vi "KeyBoardSimulation.vi"() -> ()   [LabVIEW 2016, in "DronaTest.lvlib" / "test_ValueSignal.lvlib"]
uses:
  test_ValueSignal.lvlib
  Helper/HelperVI-keyboardsimulation.vi
  main/apis/Setup/GetVI/GetVIByPath.vi
  main/apis/Assert/AssertControlValue/Equal.vi
  main/apis/Assert/AssertControlValue/True.vi
  main/apis/Stimulus/ValueSignal/ValueSignalByPathString.vi
  main/Drona.lvlib
  main/apis/Setup/GetVI/GetVI.lvlib
  main/apis/Assert/AssertControlValue/AssertControlValue.lvlib
  <vilib>/addons/_JKI Toolkits/Caraya/classes/Test/Test.lvclass
  main/apis/Stimulus/ValueSignal/ValueSignal.lvlib
panel:
  out "error out":errorcluster
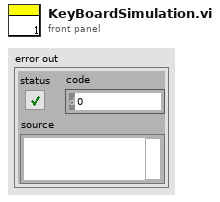
[diagram p1: front panel]
types:
  T1 = cluster{" Key":u8, "Action":enum16{"Press", "Up", "Down"}, "Delay (ms)":u32}[]
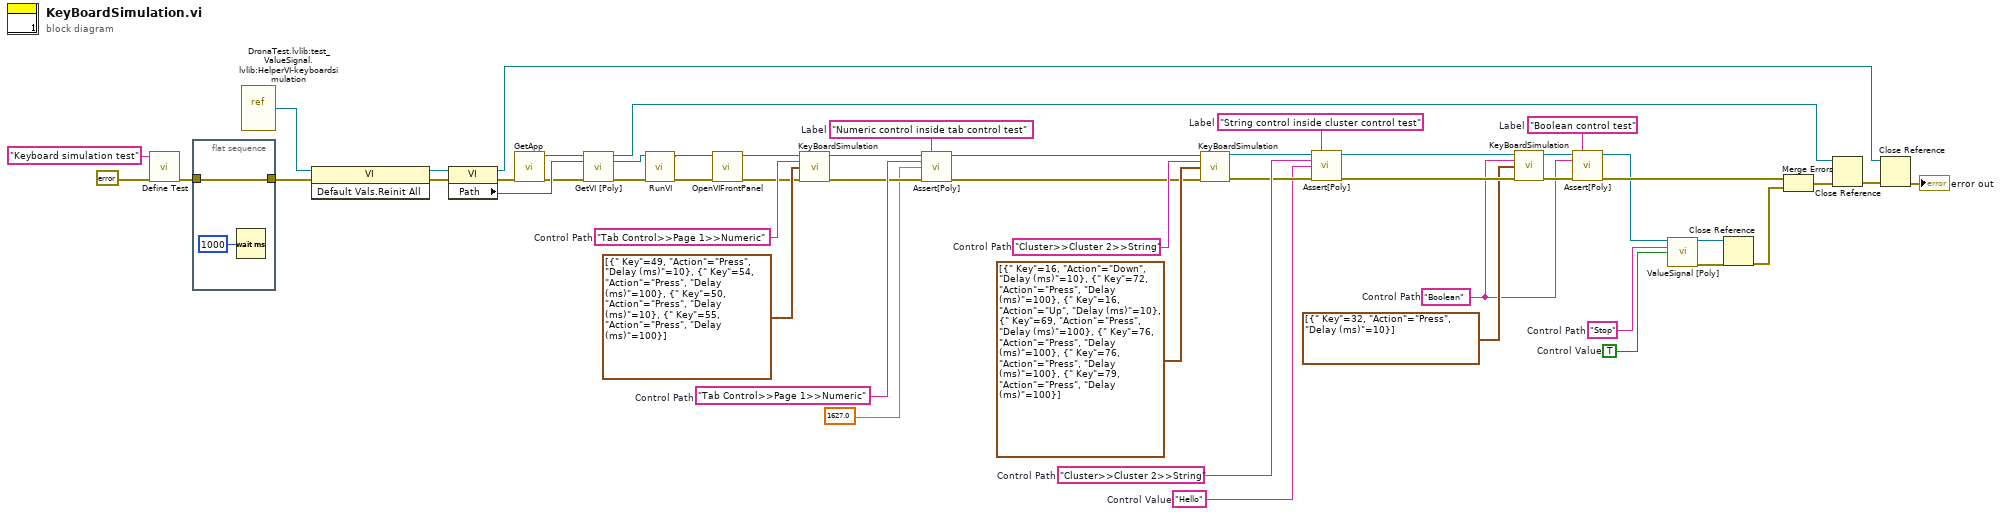
[diagram p0: block diagram]
diagram:
  w1 = "Boolean control test"  # Label
  w2 = "Boolean"  # Control Path
  w27 = TRUE  # Control Value
  w28 = "Stop"  # Control Path
  w30 = "Hello"  # Control Value
  w35 = "String control inside cluster control test"  # Label
  w36 = "Cluster>>Cluster 2>>String"  # Control Path
  w38 = "Tab Control>>Page 1>>Numeric"  # Control Path
  w43 = "Numeric control inside tab control test"  # Label
  w44 = "Tab Control>>Page 1>>Numeric"  # Control Path
  w32 = "Cluster>>Cluster 2>>String"  # Control Path
  n1 = call <vilib>:"Define Test.vi"("error in (no error)"=errorcluster {"status"=FALSE, "code"=0, "source"=""}, "Label (VI Title)"="Keyboard simulation test") -> ("error out"=w15:errorcluster)  [unwired: 9 in]
  n2 = flat-sequence {
    tunnel: w15 -> [w54]
    tunnel: [w54] -> w14
    frame #0 {
      n3 = Wait (ms)(milliseconds to wait=u32 1000) -> ()  [unwired: 1 out]
    }
  }
  n4 = vi-ref "DronaTest.lvlib:test_ValueSignal.lvlib:HelperVI-keyboardsimulation.vi"() -> (w18:refnum<vi>)
  n5 = invoke class="VI" method="Default Vals.Reinit All"(reference=w18, error in=w14) -> (reference out=w19:refnum<vi>, error out=w20:errorcluster)  [unwired: 1 in, 1 out]
  n6 = property on="Property Node" class="VI"(reference=w19, error in=w20) -> (reference out=w45:refnum<vi>, error out=w49:errorcluster, "Path"=w48:path)
  n7 = call "GetApp.vi"("error in (no error)"=w49) -> ("Application Ref"=w50:refnum<vi>, "error out"=w47:errorcluster)  [unwired: 13 in]
  n8 = call-poly "GetVI [Poly].vi"("Application Ref in"=w50, "VI Path"=w48, "error in (no error)"=w47) -> ("Application Ref out"=w46:refnum<vi>, "VI Reference"=w41:refnum<vi>, "error out"=w42:errorcluster)  [unwired: 10 in]
  n9 = call "RunVI.vi"("VI Reference In"=w41, "error in"=w42) -> ("VI Reference Out"=w12:refnum<vi>, "error out"=w13:errorcluster)  [unwired: 12 in]
  n10 = call "OpenVIFrontPanel.vi"("VI Reference In"=w12, "error in"=w13) -> ("VI Reference Out"=w11:refnum<vi>, "error out"=w10:errorcluster)  [unwired: 12 in]
  n11 = call "KeyBoardSimulation.vi"("VI Reference In"=w11, "Control Path"=w38, "Key Array"=T1 [{" Key"=49, "Action"=enum."Press", "Delay (ms)"=10}, {" Key"=54, "Action"=enum."Press", "Delay (ms)"=100}, {" Key"=50, "Action"=enum."Press", "Delay (ms)"=10}, {" Key"=55, "Action"=enum."Press", "Delay (ms)"=100}], "error In"=w10) -> ("VI Reference Out"=w39:refnum<vi>, "error IO"=w40:errorcluster)  [unwired: 10 in]
  n12 = call-poly "Assert[Poly].vi"("VI Reference In"=w39, "Label"=w43, "Control Path"=w44, "Control Value"=1627.0, "Error In"=w40) -> ("VI Reference Out"=w24:refnum<vi>, "Error Out"=w25:errorcluster)  [unwired: 9 in]
  n13 = call "KeyBoardSimulation.vi"("VI Reference In"=w24, "Control Path"=w32, "Key Array"=T1 [{" Key"=16, "Action"=enum."Down", "Delay (ms)"=10}, {" Key"=72, "Action"=enum."Press", "Delay (ms)"=100}, {" Key"=16, "Action"=enum."Up", "Delay (ms)"=10}, {" Key"=69, "Action"=enum."Press", "Delay (ms)"=100}, {" Key"=76, "Action"=enum."Press", "Delay (ms)"=100}, {" Key"=76, "Action"=enum."Press", "Delay (ms)"=100}, {" Key"=79, "Action"=enum."Press", "Delay (ms)"=100}], "error In"=w25) -> ("VI Reference Out"=w33:refnum<vi>, "error IO"=w34:errorcluster)  [unwired: 10 in]
  n14 = call-poly "Assert[Poly].vi"("VI Reference In"=w33, "Label"=w35, "Control Path"=w36, "Control Value"=w30, "Error In"=w34) -> ("VI Reference Out"=w8:refnum<vi>, "Error Out"=w9:errorcluster)  [unwired: 9 in]
  n15 = call "KeyBoardSimulation.vi"("VI Reference In"=w8, "Control Path"=w2, "Key Array"=T1 [{" Key"=32, "Action"=enum."Press", "Delay (ms)"=10}], "error In"=w9) -> ("VI Reference Out"=w4:refnum<vi>, "error IO"=w6:errorcluster)  [unwired: 10 in]
  n16 = call-poly "Assert[Poly].vi"("VI Reference In"=w4, "Label"=w1, "Control Path"=w2, "Error In"=w6) -> ("VI Reference Out"=w3:refnum<vi>, "Error Out"=w5:errorcluster)  [unwired: 10 in]
  n17 = call-poly "ValueSignal [Poly].vi"("VI Reference In"=w3, "Control Path"=w28, "Value (Signaling)"=w27) -> ("VI Reference Out"=w26:refnum<vi>, "error out"=w23:errorcluster)  [unwired: 11 in]
  n18 = Close Reference(reference=w26, error in (no error)=w23) -> (error out=w21:errorcluster)
  n19 = Merge Errors(w5, w21) -> (w22:errorcluster)
  n20 = Close Reference(reference=w46, error in (no error)=w22) -> (error out=w52:errorcluster)
  n21 = Close Reference(reference=w45, error in (no error)=w52) -> (error out=→"error out":errorcluster)
